vi "Shoot(Manual).vi"(5 "CollectSpeed(t/100ms)":dbl, 6 "Joystick":dbl, 7 "LaunchSpeed(t/100ms)":dbl, 8 "error in":errorcluster, 9 "Collection Trigger":bool, 10 "Spinup Trigger":bool, 11 "Trigger":bool) -> (0 "error out":errorcluster)   [LabVIEW 2015]
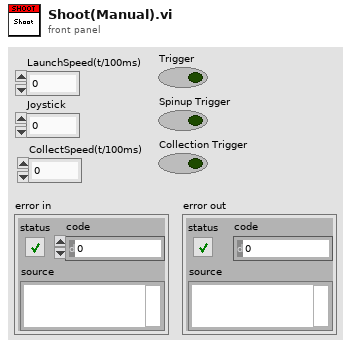
[diagram p1: front panel]
types:
  T1 = typedef "Bundle.ctl" = cluster{"TopHallRefnum":T2, "BottomHallRefnum":T2, "error":errorcluster, "LeftWheelRefnum":T4, "RightWheelRefnum":T4, "PushSolenoidRefnum":T11, "AngleMotorPosition(t)":dbl, "LaunchSpeed(t/100ms)":dbl, "CollectSpeed(t/100ms)":dbl, "SpinupDuration(10ms)":i32, "ShotDuration(10ms)":i32, "PowerScale":dbl, "AngleShift":i32, "VisionPrepAngle":dbl}
  T2 = typedef "WPI_DigitalInputDevRef.ctl" = cluster{"DevStatus":errorcluster, "DIO Channel":T3}
  T3 = typedef "FPGA_DIOChannel.ctl" = enum8{"DIO 0", "DIO 1", "DIO 2", "DIO 3", "DIO 4", "DIO 5", "DIO 6", "DIO 7", "DIO 8", "DIO 9", "DIO MXP 0", "DIO MXP 1", "DIO MXP 2", "DIO MXP 3", "DIO MXP 4", "DIO MXP 5", "DIO MXP 6", "DIO MXP 7", "DIO MXP 8", "DIO MXP 9", "DIO MXP 10", "DIO MXP 11", "DIO MXP 12", "DIO MXP 13", "DIO MXP 14", "DIO MXP 15", "Invalid"}
  T4 = typedef "WPI_MotorControlDeviceRef.ctl" = cluster{"DeviceStatus":errorcluster, "Type":T5, "PWM":cluster{"PWM Channel":T6, "DeadBand":T7}, "CAN":cluster{"Device Number":u8, "Control Mode":T8, "Semaphore":T9, "Max Vout":dbl, "TalonSRX Control Mode":T10}, "Invert":bool}
  T5 = typedef "WPI_MotorControlType.ctl" = enum16{"PWM", "CAN", "CANTalonSRX"}
  T6 = typedef "FPGA_DIOPWMChannel.ctl" = enum8{"PWM 0", "PWM 1", "PWM 2", "PWM 3", "PWM 4", "PWM 5", "PWM 6", "PWM 7", "PWM 8", "PWM 9", "PWM MXP 0", "PWM MXP 1", "PWM MXP 2", "PWM MXP 3", "PWM MXP 4", "PWM MXP 5", "PWM MXP 6", "PWM MXP 7", "PWM MXP 8", "PWM MXP 9", "Invalid"}
  T7 = typedef "WPI_PWMDeadband.ctl" = cluster{"Name":string, "maxPositivePwm":i32, "minPositivePwm":i32, "centerPwm":i32, "maxNegativePwm":i32, "minNegativePwm":i32, "angularRange":u16}
  T8 = typedef "WPI_CANJaguar_ControlMode.ctl" = enum8{"Percent VBus", "Current", "Speed", "Position", "Voltage"}
  T9 = typedef "Semaphore RefNum" = refnum<k1>
  T10 = typedef "WPI_CANTalonSRX_APIControlMode.ctl" = enum8{"Percent VBus", "Speed", "Position", "Slave", "Unchanged / Invalid", "Voltage Compensation", "Current", "Motion Profile"}
  T11 = typedef "WPI_SolenoidDevRef.ctl" = cluster{"DevStatus":errorcluster, "Pneumatics Control Module":u8, "Forward Solenoid Channel":T12, "Reverse Solenoid Channel":T12}
  T12 = typedef "WPI_SolenoidChannel.ctl" = enum8{"Solenoid 0", "Solenoid 1", "Solenoid 2", "Solenoid 3", "Solenoid 4", "Solenoid 5", "Solenoid 6", "Solenoid 7", "Invalid"}
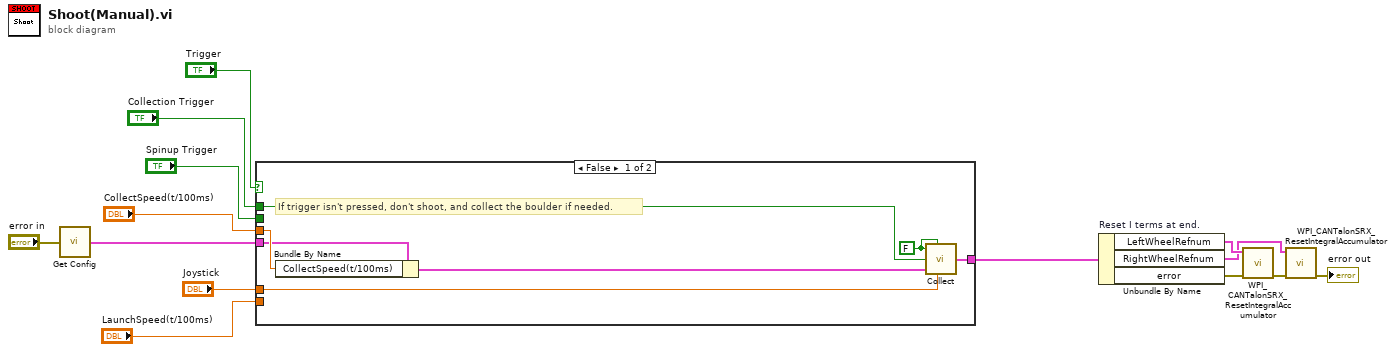
[diagram p0: block diagram]
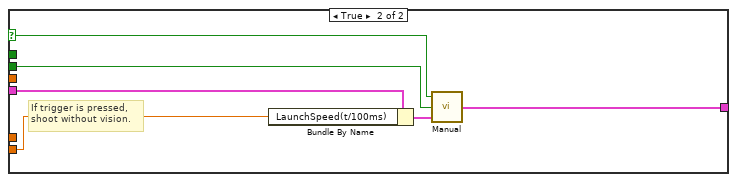
[diagram p2: hidden frame]
diagram:
  n1 = call "Get Config.vi"("error in"="error in") -> (0:w3:T1)
  n2 = case shown="False" "Trigger" {
    selector: "Trigger" -> [_ w26]
    tunnel: w3 -> [w18 w27]
    tunnel: [w20 w22] -> w2
    tunnel: "Collection Trigger" -> [w21 _]
    tunnel: "Spinup Trigger" -> [_ w25]
    tunnel: "LaunchSpeed(t/100ms)" -> [_ w24]
    tunnel: "Joystick" -> [w15 _]
    tunnel: "CollectSpeed(t/100ms)" -> [w19 _]
    frame False {
      w16 = FALSE ("VisionPrepButton")
      # "If trigger isn't pressed, don't shoot, and collect the boulder if needed."
      n3 = Bundle By Name(cluster=w18, "CollectSpeed(t/100ms)"=w19) -> (w17:T1)
      n4 = call "Collect.vi"("LowerButton"=w16, "VisionPrepButton"=w16, "CollectionTrigger"=w21, "Firing Data"=w17, "Joystick"=w15) -> ("Firing Data"=w20:T1)
    }
    frame True {
      # "If trigger is pressed,\nshoot without vision."
      n5 = Bundle By Name(cluster=w27, "LaunchSpeed(t/100ms)"=w24) -> (w23:T1)
      n6 = call "Manual.vi"("Firing Data"=w23, "Spinup Trigger"=w25, "Trigger"=w26) -> ("output cluster"=w22:T1)
    }
  }
  n7 = Unbundle By Name "Reset I terms at end."(w2) -> ("LeftWheelRefnum"=w12:T4, "RightWheelRefnum"=w11:T4, "error"=w1:errorcluster)
  n8 = call <vilib>:"WPI_CANTalonSRX_ResetIntegralAccumulator.vi"("error in (no error)"=w1, "CAN Talon SRX Ref"=w12) -> ("error out"=w14:errorcluster)  [unwired: 8 in, 1 out]
  n9 = call <vilib>:"WPI_CANTalonSRX_ResetIntegralAccumulator.vi"("error in (no error)"=w14, "CAN Talon SRX Ref"=w11) -> ("error out"=→"error out":errorcluster)  [unwired: 8 in, 1 out]
